vi "GetSetFixModeCommand.vi"() -> (3 "Command":u8[](array[numeric]) format="%x")   [LabVIEW 2017]
uses:
  <instrlib>/Samwontech TEMP2xxx/Samwontech TEMP2xxx.lvlib
panel:
  out "Command":string
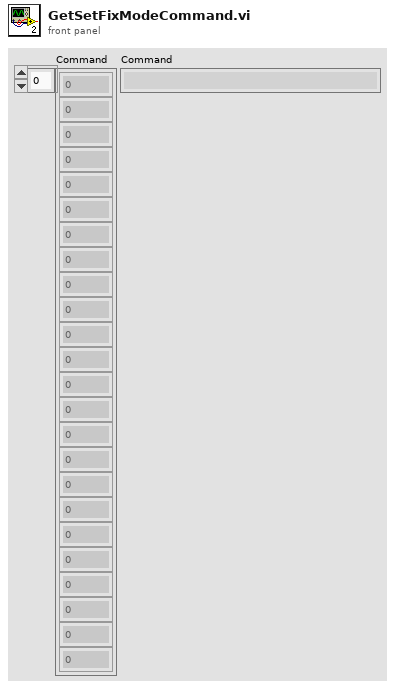
[diagram p1: front panel]
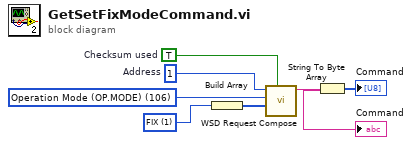
[diagram p0: block diagram]
diagram:
  w6 = u8 1  # Address
  w7 = TRUE  # Checksum used
  w4 = u32 1 items=["PROG", "FIX"] ("Operation Mode")
  w5 = u32 106 items=["Current PV (NPV)"=1, "Operation Control (COM.OPMODE)"=102, "Set Point on FIX operation (FIX.TSP)"=104, "Operation Mode (OP.MODE)"=106] ("D-Registers Map")
  n1 = Build Array(w4) -> (w3:u32[])
  n2 = call <instrlib>:"WSD Request Compose.vi"("Checksum used"=w7, "Data"=w3, "D-register number"=w5, "Address"=w6) -> ("Request"=w2:string)  [unwired: 6 in, 1 out]
  "Command" <- w2
  n3 = String To Byte Array(string=w2) -> (unsigned byte array=→"Command":u8[])
